vi "ACC_LabVIEW_BuildEmptyString.vi"(1 "Length":u32) -> (0 "String":string)   [LabVIEW 2014, in "ACC_LabVIEW.lvlib"]
doc: "generates an empty string of the given length."
uses:
  ACC_LabVIEW.lvlib
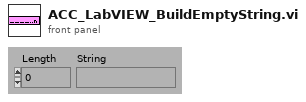
[diagram p1: front panel]
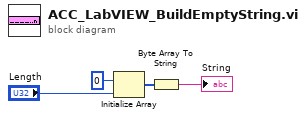
[diagram p0: block diagram]
diagram:
  n1 = Initialize Array(u8 0, "Length") -> (w2:u8[])
  n2 = Byte Array To String(unsigned byte array=w2) -> (string=→"String":string)
